vi "LoadController.vi"(8 "error in (no error)":errorcluster, 10 "Actor In":refnum<class "Actor.lvclass">, 11 "DemoStepMotor in":refnum<class "DemoStepMotor.lvclass">) -> (0 "error out":errorcluster, 3 "DemoStepMotor out":refnum<class "DemoStepMotor.lvclass">)   [LabVIEW 2020, in "DemoStepMotor.lvlib" / "DemoStepMotor.lvclass"]
uses:
  DemoStepMotor.lvclass
  ViewController/StepMotorController/StepMotorController.lvclass
  Hardware Abstraction Layer/Component/Stage/Stage/Stage.lvclass
  C:/Program Files/National Instruments/LabVIEW 2020/vi.lib/ActorFramework/Actor/Actor.lvclass
  <vilib>/ActorFramework/Actor/Actor.lvclass
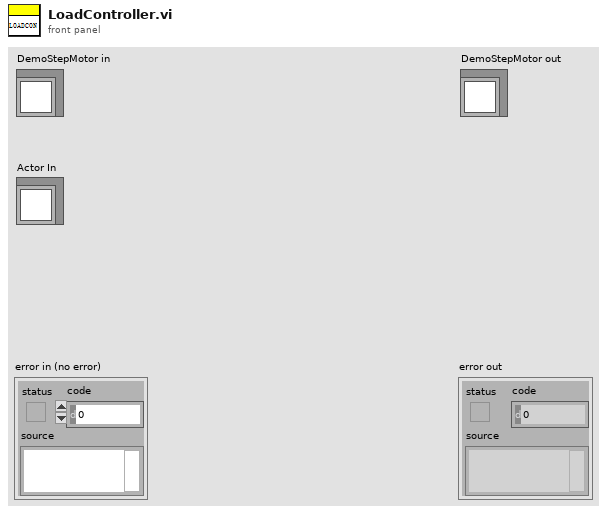
[diagram p1: front panel]
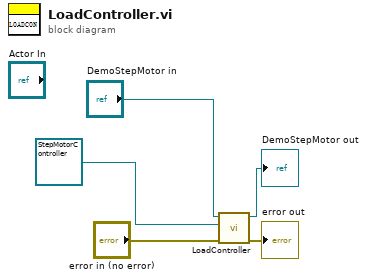
[diagram p0: block diagram]
diagram:
  n1 = call-parent "LoadController.vi"("error in (no error)"="error in (no error)", "Actor In"=refnum<class "StepMotorController.lvclass"> refnum ("StepMotorController.lvlib:StepMotorController.lvclass"), "Device in"="DemoStepMotor in") -> ("error out"=→"error out":errorcluster, "Device out"=→"DemoStepMotor out":refnum<class "DemoStepMotor.lvclass">)  [unwired: 7 in]
